vi "Set Inductance.vi"(2 "error in":T1, 3 "Magnet Inductance (H)":dbl format="%.3f", 4 "connection ID":refnum<visa-resource-name>) -> (0 "error out":T1, 1 "connection ID out":refnum<visa-resource-name>)   [LabVIEW 2019]
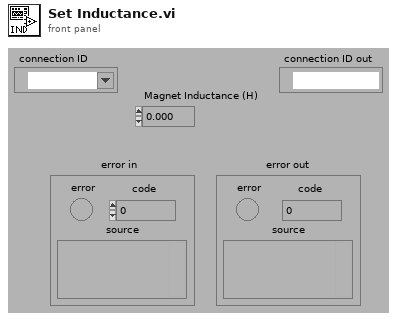
[diagram p1: front panel]
types:
  T1 = cluster{"error":bool, "code":i32, "source":string}
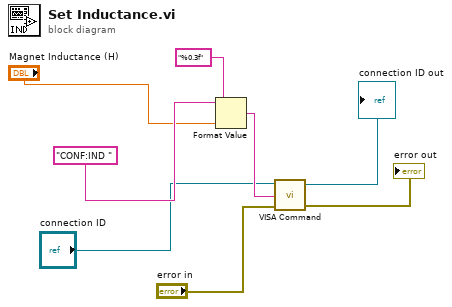
[diagram p0: block diagram]
diagram:
  n1 = Format Value(string ("")="CONF:IND ", format string="%0.3f", value (0)="Magnet Inductance (H)") -> (output string=w5:string)
  n2 = call "VISA Command.vi"("error in (no error)"="error in", "Command"=w5, "VISA resource name"="connection ID") -> ("error out"=→"error out":errorcluster, "VISA resource name out"=→"connection ID out":refnum<visa-resource-name>)  [unwired: 1 in, 1 out]
